vi "Do WS Action.vi"(4 "Secret ID (Default)":string, 5 "WS Name":string, 6 "Access ID (Default)":string, 7 "Action":T1, 8 "error in (no error)":errorcluster, 9 "Port":u16, 10 "Host":string, 11 "Scheme (HTTP)":T2) -> (0 "error out":errorcluster)   [LabVIEW 2020, in "WS Admin.lvlib"]
uses:
  WS Admin.lvlib
  Scheme.ctl
  WS Action.ctl
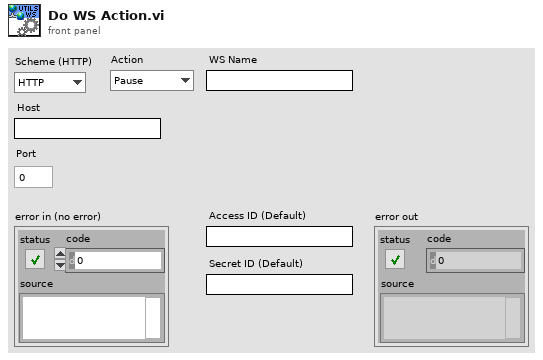
[diagram p1: front panel]
types:
  T1 = typedef "WS Admin.lvlib/WS Action.ctl" = enum16{"Pause", "Resume", "Restart", "Unpublish"}
  T2 = typedef "WS Admin.lvlib/Scheme.ctl" = enum16{"HTTP", "HTTPS"}
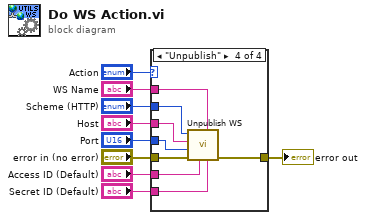
[diagram p0: block diagram]
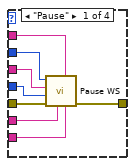
[diagram p2: hidden frame]
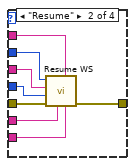
[diagram p3: hidden frame]
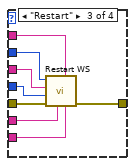
[diagram p4: hidden frame]
diagram:
  n1 = case shown="\"Unpublish\"" "Action" {
    tunnel: "error in (no error)" -> [w17 w25 w33 w41]
    tunnel: "Port" -> [w16 w20 w30 w37]
    tunnel: "Host" -> [w15 w21 w31 w38]
    tunnel: "Scheme (HTTP)" -> [w14 w22 w32 w39]
    tunnel: "WS Name" -> [w13 w23 w29 w40]
    tunnel: "Access ID (Default)" -> [w12 w19 w28 w36]
    tunnel: "Secret ID (Default)" -> [w11 w18 w27 w35]
    tunnel: [w10 w24 w26 w34] -> w1
    frame "Pause" {
      n2 = call "Pause WS.vi"("Secret ID (Default)"=w11, "WS Name"=w13, "Access ID (Default)"=w12, "error in (no error)"=w17, "Port"=w16, "Host"=w15, "Scheme (HTTP)"=w14) -> ("error out"=w10:errorcluster)  [unwired: 4 in]
    }
    frame "Resume" {
      n3 = call "Resume WS.vi"("Secret ID (Default)"=w18, "WS Name"=w23, "Access ID (Default)"=w19, "error in (no error)"=w25, "Port"=w20, "Host"=w21, "Scheme (HTTP)"=w22) -> ("error out"=w24:errorcluster)  [unwired: 4 in]
    }
    frame "Restart" {
      n4 = call "Restart WS.vi"("Secret ID (Default)"=w27, "WS Name"=w29, "Access ID (Default)"=w28, "error in (no error)"=w33, "Port"=w30, "Host"=w31, "Scheme (HTTP)"=w32) -> ("error out"=w26:errorcluster)  [unwired: 4 in]
    }
    frame "Unpublish" {
      n5 = call "Unpublish WS.vi"("Secret ID (Default)"=w35, "WS Name"=w40, "Access ID (Default)"=w36, "error in (no error)"=w41, "Port"=w37, "Host"=w38, "Scheme (HTTP)"=w39) -> ("error out"=w34:errorcluster)  [unwired: 4 in]
    }
  }
  "error out" <- w1
